vi "take_str_from_BSON_bytes.vi"(11 "BSONbytes":u8[](array[numeric]) format="%02d") -> (2 "restOfBytes":u8[](array[numeric]), 3 "value":string)   [LabVIEW 2015, in "BSON_convertors_Library.lvlib"]
doc: "Created by Artem Shevelev\nLabVIEW Portal profile: http://www.labviewportal.org/memberlist.php?mode=viewprofile&u=2340\ne-mail: artem.sh@gmail.com\nshevelev.pro"
uses:
  BSON_convertors_Library.lvlib
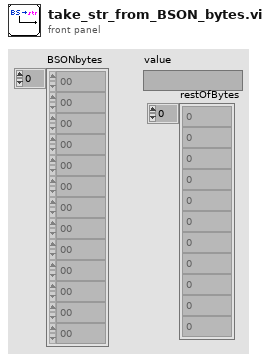
[diagram p1: front panel]
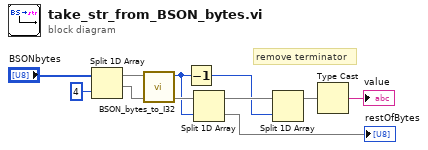
[diagram p0: block diagram]
diagram:
  # "remove terminator"
  n1 = Split 1D Array(array="BSONbytes", index=4 ("length")) -> (first subarray=w7:u8[], second subarray=w6:u8[])
  n2 = call "BSON_bytes_to_I32.vi"("BSONbytes"=w7) -> ("value"=w5:i32)  [unwired: 10 in]
  n3 = Decrement(x=w5) -> (x-1=w3:i32)
  n4 = Split 1D Array(array=w6, index=w5) -> (first subarray=w4:u8[], second subarray=→"restOfBytes":u8[])
  n5 = Split 1D Array(array=w4, index=w3) -> (first subarray=w2:u8[])  [unwired: 1 out]
  n6 = Type Cast(x=w2) -> (*(type *) &x=→"value":string)  [unwired: 1 in]
